vi "Configure Data Storage.vi"(8 "error in (no error)":errorcluster, 9 "Operation (0: Load Data Pattern)":i32(ring) items=["Load Data Pattern", "Load Bit Shape Waveform", "Store Data Pattern", "Store Bit Shape Waveform"], 10 "Data Name ()":string, 11 "VISA resource name":refnum<visa-resource-name>) -> (0 "error out":errorcluster, 3 "VISA resource name out":refnum<visa-resource-name>)   [LabVIEW 2009, in "Agilent 81150.lvlib"]
doc: "Loads or stores pattern data."
uses:
  Agilent 81150.lvlib
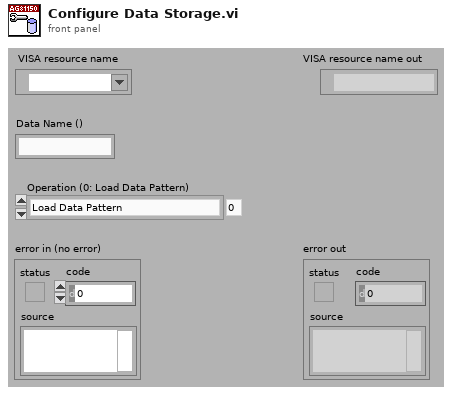
[diagram p1: front panel]
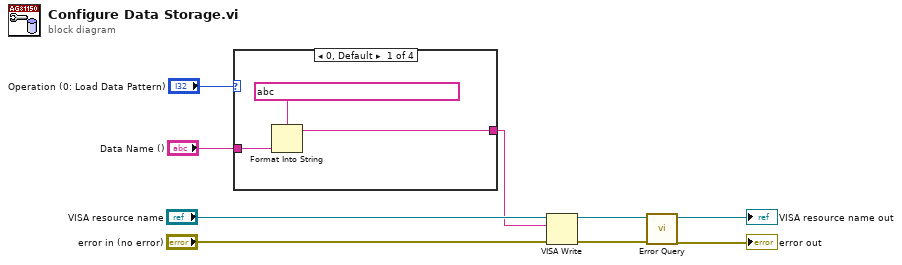
[diagram p0: block diagram]
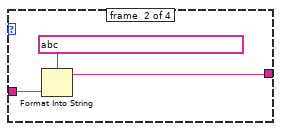
[diagram p2: hidden frame]
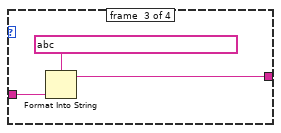
[diagram p3: hidden frame]
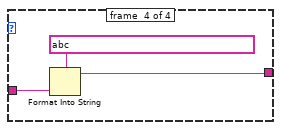
[diagram p4: hidden frame]
diagram:
  n1 = case shown="0, Default" "Operation (0: Load Data Pattern)" {
    tunnel: "Data Name ()" -> [w12 w15 w18 w21]
    tunnel: [w10 w13 w16 w19] -> w1
    frame #0 {
      n2 = Format Into String(format string=string ?, w12) -> (resulting string=w10:string)  [unwired: 2 in, 1 out]
    }
    frame #1 {
      n3 = Format Into String(format string=string ?, w15) -> (resulting string=w13:string)  [unwired: 2 in, 1 out]
    }
    frame #2 {
      n4 = Format Into String(format string=string ?, w18) -> (resulting string=w16:string)  [unwired: 2 in, 1 out]
    }
    frame #3 {
      n5 = Format Into String(format string=string ?, w21) -> (resulting string=w19:string)  [unwired: 2 in, 1 out]
    }
  }
  n6 = VISA Write(VISA resource name="VISA resource name", write buffer=w1, error in (no error)="error in (no error)") -> (VISA resource name out=w7:refnum<visa-resource-name>, error out=w6:errorcluster)  [unwired: 1 out]
  n7 = call "Error Query.vi"("error in (no error)"=w6, "VISA resource name"=w7) -> ("error out"=→"error out":errorcluster, "VISA resource name out"=→"VISA resource name out":refnum<visa-resource-name>)  [unwired: 6 in, 2 out]
